vi "Set Line Interlock Configuration.vi"(8 "error in (no error)":errorcluster, 9 "Manual Mode (False)":bool, 10 "Bit Field In":u16, 11 "Storage Line in":refnum<class "Storage Line.lvclass">) -> (0 "error out":errorcluster, 1 "Interlock Chain out":refnum<class "Interlock Chain.lvclass">, 2 "Bit Field out":u16, 3 "Storage Line out":refnum<class "Storage Line.lvclass">)   [LabVIEW 2015, in "cRIO-Carbondioxide.lvlib" / "CO2-Actor.lvlib" / "Storage Line.lvclass"]
uses:
  Storage Line.lvclass
  Interlocks/Interlock Chain/Interlock Chain.lvclass
  Interlocks/Interlock/Interlock.lvclass
  Interlocks/Controls/Add IL to -Enumerator.ctl
  Transfer Line/Transfer Line.lvclass
  Interlocks/Interlock Sample/Interlock Sample.lvclass
  subs/Sample/Sample.lvclass
  Storage Line.lvclass/Storage Line.ctl
  CO2 Actor Messages/Ping Msg/Ping Msg.lvclass/Ping Msg.ctl
  <vilib>/ActorFramework/Message Enqueuer/Message Enqueuer.lvclass/Message Enqueuer.ctl
  Transfer Line/Transfer Line.lvclass/Transfer Line.ctl
  Interlocks/Interlock U16/Seize/IL U16 Seize.lvclass
  Interlocks/Interlock U16/Seize/IL U16 Seize.lvclass/IL U16 Seize.ctl
  Interlocks/Interlock Chain/Interlock Chain.lvclass/Interlock Chain.ctl
  <vilib>/ActorFramework/Message Enqueuer/Enqueue.vi
  <vilib>/ActorFramework/Message Priority Queue/Priority Enqueue.vi
  subs/Sample/Read Sample From Container.vi
  CO2 Actor Messages/Ping Msg/Ping Msg.lvclass
  <vilib>/ActorFramework/Actor/Actor.lvclass
  CO2 Actor/CO2 Actor.lvclass
  cRIO-CO2/cRIO-CO2.lvclass
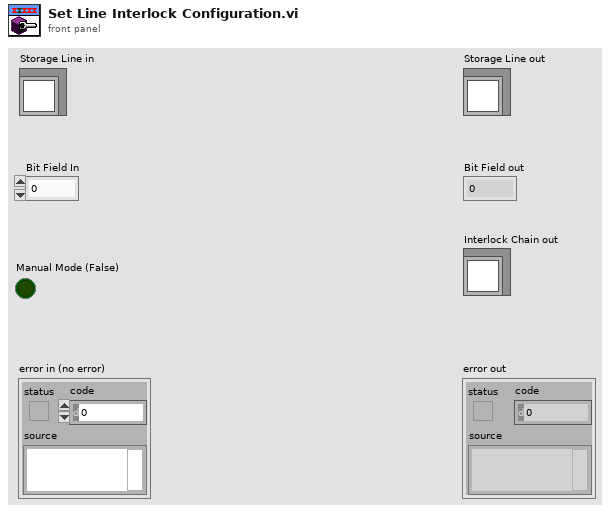
[diagram p1: front panel]
types:
  T1 = typedef "Add IL to -Enumerator.ctl" = enum16{"Deny", "Allow", "None"}
  T2 = typedef "Dedicated Enqueuers.ctl" = cluster{"Freezers":cluster{"Syringe":refnum<class "Message Enqueuer.lvclass">, "Tank 1":refnum<class "Message Enqueuer.lvclass">, "Tank 2":refnum<class "Message Enqueuer.lvclass">, "Tank 3":refnum<class "Message Enqueuer.lvclass">, "Tank 4":refnum<class "Message Enqueuer.lvclass">}, "Heaters":cluster{"Syringe":refnum<class "Message Enqueuer.lvclass">, "Piston":refnum<class "Message Enqueuer.lvclass">}, "Blowers":cluster{"Tank 1":refnum<class "Message Enqueuer.lvclass">, "Tank 2":refnum<class "Message Enqueuer.lvclass">, "Tank 3":refnum<class "Message Enqueuer.lvclass">, "Tank 4":refnum<class "Message Enqueuer.lvclass">, "Syringe":refnum<class "Message Enqueuer.lvclass">}, "Sample Line":refnum<class "Message Enqueuer.lvclass">, "Storage Line":refnum<class "Message Enqueuer.lvclass">, "Transfer Line":refnum<class "Message Enqueuer.lvclass">, "Syringe Stepper":refnum<class "Message Enqueuer.lvclass">, "Syringe Line":refnum<class "Message Enqueuer.lvclass">, "Capillary Line":refnum<class "Message Enqueuer.lvclass">, "Preparation Line":refnum<class "Message Enqueuer.lvclass">, "Turbo":refnum<class "Message Enqueuer.lvclass">, "Vacuum":refnum<class "Message Enqueuer.lvclass">, "He Line":refnum<class "Message Enqueuer.lvclass">, "Cylinder":refnum<class "Message Enqueuer.lvclass">}
  T3 = typedef "Sample Container.ctl" = cluster{"Sample In":refnum<k21>, "Sample Name":refnum<k21>, "Ti Cathode":refnum<k21>, "SampleQ":refnum<queue>}
  T4 = typedef "Sample Transfer Container Enumerator.ctl" = enum16{"None", "Sample 1", "Sample 2", "Sample 3", "Sample 4", "Sample 5", "Storage 01", "Storage 02", "Storage 03", "Storage 04", "Storage 05", "Storage 06", "Storage 07", "Storage 08", "Storage 09", "Storage 10", "Storage 11", "Storage 12", "Syringe", "Undefined"}
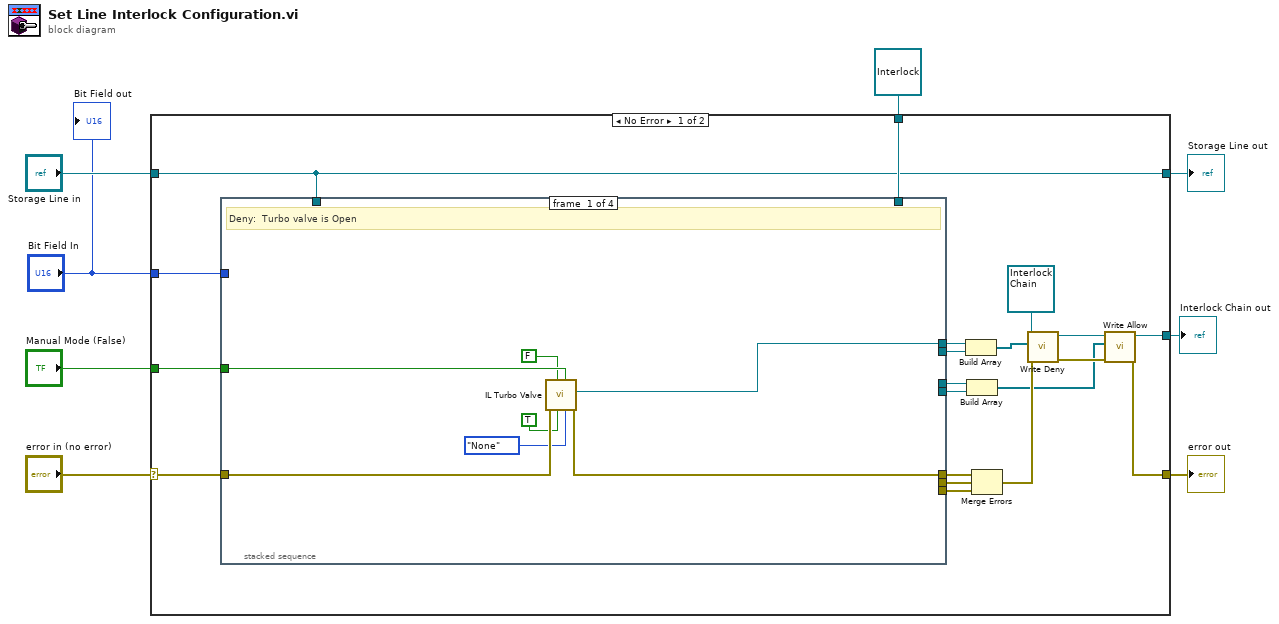
[diagram p0: block diagram]
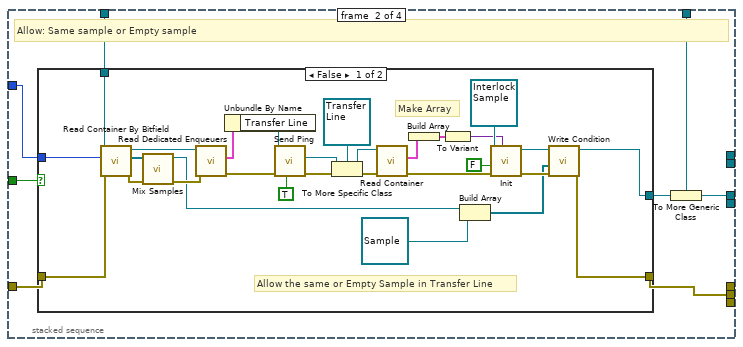
[diagram p2: hidden frame]
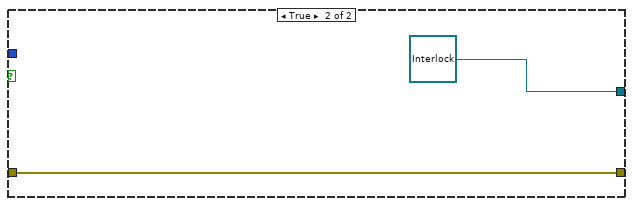
[diagram p3: hidden frame]
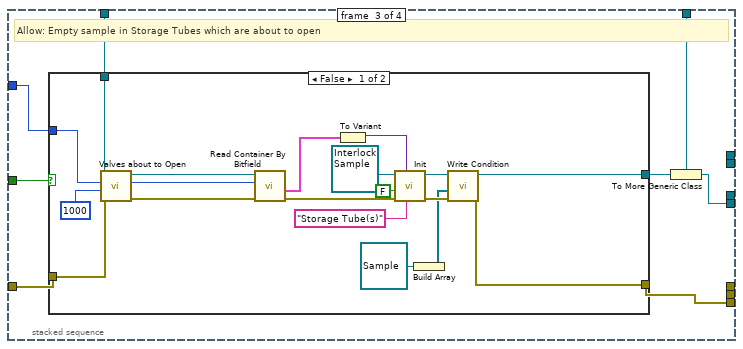
[diagram p4: hidden frame]
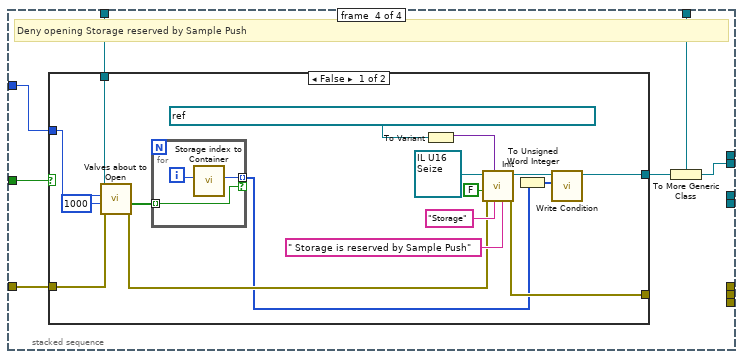
[diagram p6: hidden frame]
diagram:
  n1 = case shown="No Error" "error in (no error)" {
    selector: "error in (no error)" -> [w28 w132]
    tunnel: [w14 w132] -> w7
    tunnel: [w20 w131] -> w5
    tunnel: "Storage Line in" -> [w20 w131]
    tunnel: [w16 _] -> w4
    tunnel: "Bit Field In" -> [w26 _]
    tunnel: "Manual Mode (False)" -> [w27 _]
    tunnel: refnum<class "Interlock.lvclass"> refnum ("Interlock.lvclass") -> [w25 _]
    frame No Error {
      n2 = stacked-sequence {
        tunnel: w28 -> [w35 w41 w79 w106]
        tunnel: [w32 _ _ _] -> w22
        tunnel: [w34 _ _ _] -> w23
        tunnel: w27 -> [w33 w40 w82 w109]
        tunnel: w26 -> [_ w43 w80 w107]
        tunnel: w25 -> [_ w36 w76 w104]
        tunnel: w20 -> [_ w42 w81 w108]
        tunnel: [_ w39 _ _] -> w18
        tunnel: [_ w37 _ _] -> w13
        tunnel: [_ _ w78 _] -> w11
        tunnel: [_ _ w75 _] -> w10
        tunnel: [_ _ _ w103] -> w9
        frame #0 {
          # "Deny:  Turbo valve is Open"
          n3 = call "IL Turbo Valve.vi"("Add to (Deny)"=Add_IL_to_-Enumerator."None", "Ignore (F)"=w33, "Interlock Condition (ON/OFF)"=TRUE, "Stop Self on IL? (T)"=FALSE, "error in (no error)"=w35) -> ("error out"=w34:errorcluster, "IL Turbo Valve"=w32:refnum<class "Interlock.lvclass">)  [unwired: 4 in, 1 out]
        }
        frame #1 {
          # "Allow: Same sample or Empty sample"
          n4 = case shown="False" w40 {
            tunnel: w43 -> [w72 _]
            tunnel: w42 -> [w71 _]
            tunnel: w41 -> [w70 w74]
            tunnel: [w47 w74] -> w39
            tunnel: [w46 refnum<class "Interlock.lvclass"> refnum ("element")] -> w38
            frame False {
              # "Make Array"
              # "Allow the same or Empty Sample in Transfer Line"
              n5 = call "Read Container By Bitfield.vi"("error in (no error)"=w70, "Bitfield"=w72, "Storage Line in"=w71) -> ("error out"=w48:errorcluster, "Samples"=w69:refnum<class "Sample.lvclass">[], "Storage Line out"=w68:refnum<class "Storage Line.lvclass">)  [unwired: 4 in, 2 out]
              n6 = call "Mix Samples.vi"("error in (no error)"=w48, "Samples In"=w69) -> ("error out"=w67:errorcluster, "Sample out"=w51:refnum<class "Sample.lvclass">)  [unwired: 6 in, 2 out]
              n7 = call "Read Dedicated Enqueuers.vi"("error in (no error)"=w67, "CO2 Actor in"=w68) -> ("error out"=w65:errorcluster, "Dedicated Enqueuers"=w66:T2)  [unwired: 6 in, 2 out]
              n8 = Unbundle By Name(w66) -> ("Transfer Line"=w64:refnum<class "Message Enqueuer.lvclass">)
              n9 = call "Send Ping.vi"("Return Self (F)"=TRUE, "error in (no error)"=w65, "Message Enqueuer"=w64) -> ("error out"=w62:errorcluster, "Actor out"=w60:refnum<class "Actor.lvclass">)  [unwired: 5 in, 2 out]
              n10 = To More Specific Class(target class=refnum<class "Transfer Line.lvclass"> refnum ("Transfer Line.lvclass"), reference=w60, error in=w62) -> (specific class reference=w58:refnum<class "Transfer Line.lvclass">, error out=w59:errorcluster)
              n11 = call "Read Container.vi"("error in (no error)"=w59, "Transfer Line in"=w58) -> ("error out"=w56:errorcluster, "Sample Container"=w55:T3)  [unwired: 5 in, 3 out]
              n12 = Build Array(w55) -> (w45:T3[])
              n13 = To Variant(anything=w45) -> (Variant=w54:variant)
              n14 = Build Array(w51, refnum<class "Sample.lvclass"> refnum ("Sample.lvclass")) -> (w50:refnum<class "Sample.lvclass">[])
              n15 = call-dynamic "Init.vi"("Sample Containers SHV (Array!)"=w54, "error in (no error)"=w56, "Stop Self on IL? (T)"=FALSE, "Interlock Sample in"=refnum<class "Interlock Sample.lvclass"> refnum ("Interlock Sample.lvclass")) -> ("error out"=w53:errorcluster, "Interlock Sample out"=w52:refnum<class "Interlock Sample.lvclass">)  [unwired: 6 in]
              n16 = call "Write Condition.vi"("error in (no error)"=w53, "Samples"=w50, "Interlock Sample in"=w52) -> ("error out"=w47:errorcluster, "Interlock Sample out"=w46:refnum<class "Interlock Sample.lvclass">)  [unwired: 7 in]
            }
            frame True {
            }
          }
          n17 = To More Generic Class(target class=w36, reference=w38) -> (generic class reference=w37:refnum<class "Interlock.lvclass">)
        }
        frame #2 {
          # "Allow: Empty sample in Storage Tubes which are about to open"
          n18 = case shown="False" w82 {
            tunnel: w81 -> [w91 _]
            tunnel: w80 -> [w85 _]
            tunnel: w79 -> [w88 w102]
            tunnel: [w93 w102] -> w78
            tunnel: [w92 _] -> w77
            frame False {
              n19 = call "Valves about to Open.vi"("error in (no error)"=w88, "timeout in ms (-1)"=1000, "Requested Bit Field"=w85, "Storage Line in"=w91) -> ("error out"=w90:errorcluster, "Bitfield of valves about to Open"=w86:u16, "Storage Line out"=w89:refnum<class "Storage Line.lvclass">)  [unwired: 4 in, 1 out]
              n20 = call "Read Container By Bitfield.vi"("error in (no error)"=w90, "Bitfield"=w86, "Storage Line in"=w89) -> ("error out"=w101:errorcluster, "Containers"=w84:T3[])  [unwired: 4 in, 3 out]
              n21 = To Variant(anything=w84) -> (Variant=w100:variant)
              n22 = call-dynamic "Init.vi"("Name (SHV Name if empty)"="Storage Tube(s)", "Sample Containers SHV (Array!)"=w100, "error in (no error)"=w101, "Stop Self on IL? (T)"=FALSE, "Interlock Sample in"=refnum<class "Interlock Sample.lvclass"> refnum ("Interlock Sample.lvclass")) -> ("error out"=w97:errorcluster, "Interlock Sample out"=w96:refnum<class "Interlock Sample.lvclass">)  [unwired: 5 in]
              n23 = Build Array(refnum<class "Sample.lvclass"> refnum ("Sample.lvclass")) -> (w94:refnum<class "Sample.lvclass">[])
              n24 = call "Write Condition.vi"("error in (no error)"=w97, "Samples"=w94, "Interlock Sample in"=w96) -> ("error out"=w93:errorcluster, "Interlock Sample out"=w92:refnum<class "Interlock Sample.lvclass">)  [unwired: 7 in]
            }
            frame True {
            }
          }
          n25 = To More Generic Class(target class=w76, reference=w77) -> (generic class reference=w75:refnum<class "Interlock.lvclass">)
        }
        frame #3 {
          # "Deny opening Storage reserved by Sample Push"
          n26 = case shown="False" w109 {
            tunnel: w108 -> [w118 _]
            tunnel: w107 -> [w116 _]
            tunnel: w106 -> [w117 w130]
            tunnel: [w119 w130] -> _
            tunnel: [w123 _] -> w105
            frame False {
              n27 = call "Valves about to Open.vi"("error in (no error)"=w117, "timeout in ms (-1)"=1000, "Requested Bit Field"=w116, "Storage Line in"=w118) -> ("error out"=w114:errorcluster, "Boolean array of valves about to Open"=w113:bool[])  [unwired: 4 in, 2 out]
              n28 = for {
                tunnel: w113 -> [w127] mode=indexing
                tunnel: [w128] -> w112 mode=indexing if=w127
                i -> [w129]
                n29 = call "Storage index to Container.vi"("Index"=w129) -> ("Container"=w128:T4)  [unwired: 10 in]
              }
              n30 = To Variant(anything=refnum<k21> "ni.var.psp://crio-carbondioxide/AMS Gas SHV/Sample Push/Source Storage" ("SHV")) -> (Variant=w126:variant)
              n31 = call-dynamic "Init.vi"("Interlock message (\" -> Interlock!\")"=" Storage is reserved by Sample Push" ("Interlock message (\" -> Interlock!\")"), "Name (SHV Name if empty)"="Storage", "SHV"=w126, "error in (no error)"=w114, "Stop Self on IL? (T)"=FALSE, "Interlock in"=refnum<class "IL U16 Seize.lvclass"> refnum ("cRIO-Carbondioxide.lvlib:IL U16 Seize.lvclass")) -> ("error out"=w119:errorcluster, "Interlock out"=w124:refnum<class "IL U16 Seize.lvclass">)  [unwired: 4 in]
              n32 = To Unsigned Word Integer(number=w112) -> (unsigned 16bit integer=w111:u16[])
              n33 = call "Write Condition.vi"("Deny"=w111, "IL U16 Deny in"=w124) -> ("IL U16 Deny out"=w123:refnum<class "IL U16 Seize.lvclass">)  [unwired: 9 in]
            }
            frame True {
            }
          }
          n34 = To More Generic Class(target class=w104, reference=w105) -> (generic class reference=w103:refnum<class "Interlock.lvclass">)
        }
      }
      n35 = Build Array(w22, w9) -> (w21:refnum<class "Interlock.lvclass">[])
      n36 = Build Array(w13, w10) -> (w12:refnum<class "Interlock.lvclass">[])
      n37 = Merge Errors(w23, w18, w11) -> (w19:errorcluster)
      n38 = call "Write Deny.vi"("error in (no error)"=w19, "Deny"=w21, "Interlock Chain in"=refnum<class "Interlock Chain.lvclass"> refnum) -> ("error out"=w15:errorcluster, "Interlock Chain out"=w17:refnum<class "Interlock Chain.lvclass">)  [unwired: 7 in]
      n39 = call "Write Allow.vi"("error in (no error)"=w15, "Allow"=w12, "Interlock Chain in"=w17) -> ("error out"=w14:errorcluster, "Interlock Chain out"=w16:refnum<class "Interlock Chain.lvclass">)  [unwired: 7 in]
    }
    frame Error {
    }
  }
  "error out" <- w7
  "Storage Line out" <- w5
  "Interlock Chain out" <- w4
  "Bit Field out" <- "Bit Field In"
